vi "CTA Calib Coeff Global.vi"() -> ()   [LabVIEW 2022 SP3]
uses:
  Ctls/Calibration data.ctl
panel:
  out "HW Calibration Cluster":T1[](array[typedef])
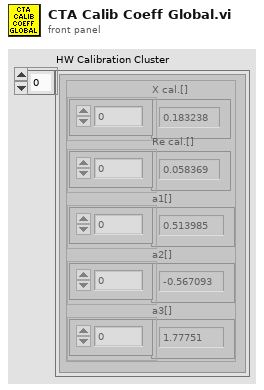
[diagram p1: front panel]
types:
  T1 = typedef "Calibration data.ctl" = cluster{"X cal.[]":dbl[], "Re cal.[]":dbl[], "a1[]":dbl[], "a2[]":dbl[], "a3[]":dbl[]}
diagram:
